vi "_Default Instrument Setup.vi"(8 "error in":errorcluster caption="error in (no error)", 11 "VISA resource name":refnum<visa-resource-name>) -> (0 "error out":errorcluster, 3 "VISA resource name out":refnum<visa-resource-name>)   [LabVIEW 2020, in "Rohde&Schwarz RTx Oscilloscopes.lvlib"]
doc: "This Utility VI sends a default command string to the instrument whenever a new VISA session is opened, or the instrument is reset.\nThis VI is intended to be used as a subVI for the Initialize.vi and Reset VI. Altering this VI could cause these two VI's to operate incorrectly."
uses:
  Rohde&Schwarz RTx Oscilloscopes.lvlib
  type_Options_Item_Parsing.ctl
  rsidr_core.lvlib
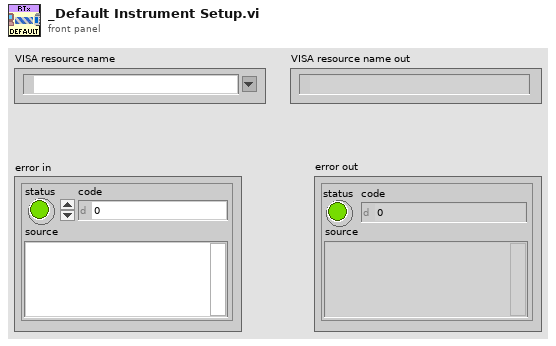
[diagram p1: front panel]
types:
  T1 = typedef "Rohde&Schwarz RTx Oscilloscopes.lvlib/rsidr_core.lvlib/type_Options_Item_Parsing.ctl" = enum16{"None", "Keep parts after dash", "Keep parts before dash", "Automatic"}
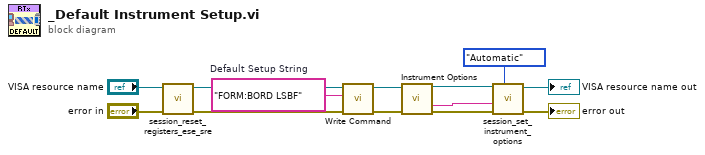
[diagram p0: block diagram]
diagram:
  w13 = "FORM:BORD LSBF"  # Default Setup String
  n1 = call "session_reset_registers_ese_sre.vi"("error in"="error in", "VISA resource name"="VISA resource name") -> ("error out"=w9:errorcluster, "VISA resource name out"=w8:refnum<visa-resource-name>)  [unwired: 8 in]
  n2 = call "Write Command.vi"("error in (no error)"=w9, "Command"=w13, "VISA resource name"=w8) -> ("error out"=w7:errorcluster, "VISA resource name out"=w6:refnum<visa-resource-name>)  [unwired: 7 in]
  n3 = call "Instrument Options.vi"("VISA resource name"=w6, "error in (no error)"=w7) -> ("VISA resource name out"=w4:refnum<visa-resource-name>, "Options List"=w12:string, "error out"=w5:errorcluster)  [unwired: 10 in, 1 out]
  n4 = call "session_set_instrument_options.vi"("Item Parsing"=type_Options_Item_Parsing."Automatic", "error in"=w5, "Options string"=w12, "VISA resource name"=w4) -> ("error out"=→"error out":errorcluster, "VISA resource name out"=→"VISA resource name out":refnum<visa-resource-name>)  [unwired: 4 in, 2 out]
